vi "Decimate 1D Array.vi"() -> ()   [LabVIEW 2015]
panel:
  out "Acceleration Data - All Channels":dbl[][](graph)
  out "Acceleration Data - Raw Data":dbl[](graph)
  in  "One Channel":dbl[](array[numeric])=[-0.14962495265155748, 0.41037504734844255, 0.7503750473484425, 1.3503750473484426, 0.32358707926196334, 0.8835870792619633, 1.2235870792619634, 1.8235870792619633, 0.5158371040723982, 1.0758371040723982, 1.4158371040723983, 2.015837104072398, 1.0013622642375388, 1.5613622642375389, 1.9013622642375387, 2.501362264237539, 1.2315810460794596, 1.7915810460794597, 2.1315810460794595, 2.7315810460794596, 1.4926225836648097, 2.0526225836648098, 2.3926225836648096, 2.9926225836648097, 1.7403663242081597, 2.30036632420816, 2.6403663242081596, 3.2403663242081597, 2.1837724556787284, 2.7437724556787284, 3.0837724556787283, 3.6837724556787284, 2.4331809540498823, 2.9931809540498824, 3.3331809540498822, 3.9331809540498823, 2.6727105780071363, 3.2327105780071363, 3.572710578007136, 4.172710578007136, 2.7527846546640786, 3.3127846546640787, 3.6527846546640785, 4.252784654664079, 3.199063134137579, 3.759063134137579, 4.099063134137579, 4.699063134137579, 3.383002482831626, 3.943002482831626, 4.283002482831626, 4.8830024828316265, 3.5393424951638277, 4.099342495163828, 4.439342495163828, 5.039342495163828, 3.678036551358494, 4.238036551358494, 4.578036551358494, 5.178036551358494, 3.77794347870013, 4.337943478700129, 4.67794347870013, 5.27794347870013, 3.972363708756191, 4.532363708756192, 4.8723637087561915, 5.472363708756191, 4.209103239125207, 4.769103239125206, 5.109103239125207, 5.709103239125207, 4.28250695958775, 4.84250695958775, 5.182506959587751, 5.78250695958775, 4.408872390322232, 4.9688723903222325, 5.308872390322232, 5.908872390322232, 4.758958504137904, 5.318958504137903, 5.658958504137904, 6.258958504137904, 4.681077878539436, 5.241077878539436, 5.581077878539436, 6.181077878539436, 4.649505296320039, 5.209505296320039, 5.5495052963200395, 6.149505296320039, 4.663003364980422, 5.223003364980421, 5.563003364980422, 6.163003364980422, 4.692743104263729, 5.252743104263729, 5.59274310426373, 6.192743104263729, 4.813363242945864, 5.373363242945864, 5.7133632429458645, 6.313363242945864, 4.8495688944798045, 5.409568894479804, 5.749568894479805, 6.3495688944798045, 4.832958271083728, 5.392958271083728, 5.732958271083729, 6.332958271083728, 4.794309425014819, 5.354309425014819, 5.694309425014819, 6.294309425014819, 4.729519768328653, 5.289519768328653, 5.629519768328653, 6.229519768328653, 4.512270957962928, 5.072270957962928, 5.412270957962928, 6.012270957962928, 4.558016333461781, 5.118016333461782, 5.4580163334617815, 6.058016333461781, 4.373550079676513, 4.933550079676513, 5.273550079676514, 5.873550079676513, 4.205404174649964, 4.765404174649964, 5.105404174649965, 5.705404174649964, 3.9620544887813622, 4.522054488781363, 4.862054488781363, 5.462054488781362, 3.9557536814065983, 4.515753681406599, 4.855753681406599, 5.455753681406598, 3.821833957543013, 4.381833957543013, 4.721833957543013, 5.321833957543014, 3.6260642782488035, 4.186064278248804, 4.526064278248803, 5.126064278248803, 3.3258171871791595, 3.8858171871791596, 4.225817187179159, 4.82581718717916, 3.0319650788286374, 3.5919650788286375, 3.9319650788286373, 4.531965078828637, 2.963344631394424, 3.523344631394424, 3.863344631394424, 4.463344631394424, 2.6667322317798274, 3.2267322317798275, 3.5667322317798273, 4.166732231779827, 2.473099379128181, 3.033099379128181, 3.3730993791281807, 3.973099379128181, 2.192699443858829, 2.752699443858829, 3.092699443858829, 3.692699443858829, 1.7970855115107007, 2.357085511510701, 2.697085511510701, 3.2970855115107005, 1.391362630806126, 1.951362630806126, 2.291362630806126, 2.891362630806126, 1.1947024580658947, 1.7547024580658948, 2.094702458065895, 2.694702458065895, 0.8293390768372463, 1.3893390768372464, 1.7293390768372463, 2.3293390768372464, 0.7165176103423602, 1.2765176103423603, 1.6165176103423602, 2.2165176103423603, 0.21739186152171264, 0.7773918615217127, 1.1173918615217127, 1.7173918615217127, 0.08389711880070679, 0.6438971188007069, 0.9838971188007068, 1.5838971188007067, -0.2014154315838475, 0.35858456841615255, 0.6985845684161525, 1.2985845684161526, -0.45880737655206777, 0.10119262344793228, 0.44119262344793225, 1.0411926234479323, -0.7588321422834481, -0.19883214228344803, 0.14116785771655194, 0.7411678577165519, -1.1726284726040646, -0.6126284726040645, -0.27262847260406453, 0.32737152739593545, -1.530929895098799, -0.970929895098799, -0.630929895098799, -0.030929895098799065, -1.855415216411067, -1.295415216411067, -0.9554152164110671, -0.3554152164110671, -2.1257997826218475, -1.5657997826218475, -1.2257997826218476, -0.6257997826218475, -2.2342862030438306, -1.6742862030438306, -1.3342862030438307, -0.7342862030438306, -2.741606398916626, -2.181606398916626, -1.841606398916626, -1.241606398916626, -2.887792759406135, -2.327792759406135, -1.987792759406135, -1.387792759406135, -3.213592959260521, -2.653592959260521, -2.313592959260521, -1.713592959260521, -3.266690568130646, -2.706690568130646, -2.3666905681306463, -1.7666905681306462, -3.6684175532113046, -3.1084175532113045, -2.7684175532113047, -2.1684175532113046, -3.8842018773676084, -3.3242018773676083, -2.9842018773676084, -2.3842018773676084, -3.7978109000808535, -3.2378109000808535, -2.8978109000808536, -2.2978109000808535, -4.162177095542973, -3.6021770955429733, -3.2621770955429734, -2.6621770955429733, -4.317899007672012, -3.757899007672012, -3.417899007672012, -2.817899007672012, -4.361940882321648, -3.8019408823216483, -3.4619408823216484, -2.8619408823216483, -4.4517483980505705, -3.8917483980505705, -3.5517483980505706, -2.9517483980505705, -4.511118204064262, -3.951118204064262, -3.611118204064262, -3.011118204064262, -4.629422702158851, -4.069422702158851, -3.729422702158851, -3.129422702158851, -4.768299148577401, -4.208299148577401, -3.868299148577401, -3.268299148577401, -4.899995619058348, -4.339995619058348, -3.9999956190583483, -3.3999956190583482, -4.766949699339253, -4.206949699339253, -3.8669496993392527, -3.2669496993392526, -4.859462074009303, -4.299462074009304, -3.9594620740093034, -3.3594620740093033, -4.852682045261981, -4.292682045261982, -3.9526820452619815, -3.3526820452619814, -4.67685667734484, -4.11685667734484, -3.7768566773448398, -3.1768566773448397, -4.690449517396064, -4.130449517396064, -3.790449517396064, -3.190449517396064, -4.8148867377571305, -4.254886737757131, -3.9148867377571306, -3.3148867377571305, -4.582687293451267, -4.022687293451266, -3.682687293451267, -3.082687293451267, -4.543532999964535, -3.983532999964535, -3.643532999964535, -3.043532999964535, -4.31781138883897, -3.7578113888389697, -3.41781138883897, -2.8178113888389698, -4.217078341071507, -3.657078341071507, -3.317078341071507, -2.717078341071507, -4.073221926285143, -3.513221926285143, -3.173221926285143, -2.573221926285143, -3.9650472381739164, -3.4050472381739163, -3.0650472381739164, -2.4650472381739164, -3.8413723612649657, -3.2813723612649657, -2.941372361264966, -2.3413723612649657, -3.617751813992966, -3.057751813992966, -2.717751813992966, -2.117751813992966, -3.342307409185613, -2.782307409185613, -2.442307409185613, -1.8423074091856129, -3.000516474277763, -2.440516474277763, -2.100516474277763, -1.500516474277763, -2.8454216030491355, -2.2854216030491354, -1.9454216030491356, -1.3454216030491355, -2.4517334968884885, -1.8917334968884885, -1.5517334968884886, -0.9517334968884885, -2.260865703872782, -1.7008657038727821, -1.3608657038727823, -0.7608657038727822, -2.1113170451710848, -1.5513170451710847, -1.2113170451710848, -0.6113170451710848, -1.8845857313028413, -1.3245857313028413, -0.9845857313028413, -0.38458573130284135, -1.4514697463196364, -0.8914697463196364, -0.5514697463196364, 0.048530253680363566, -1.2085104708975833, -0.6485104708975833, -0.3085104708975833, 0.29148952910241666, -1.0396797084617442, -0.4796797084617441, -0.13967970846174416, 0.4603202915382558, -0.5479193060350005, 0.012080693964999556, 0.3520806939649995, 0.9520806939649995, -0.30307056326094645, 0.2569294367390536, 0.5969294367390536, 1.1969294367390535]
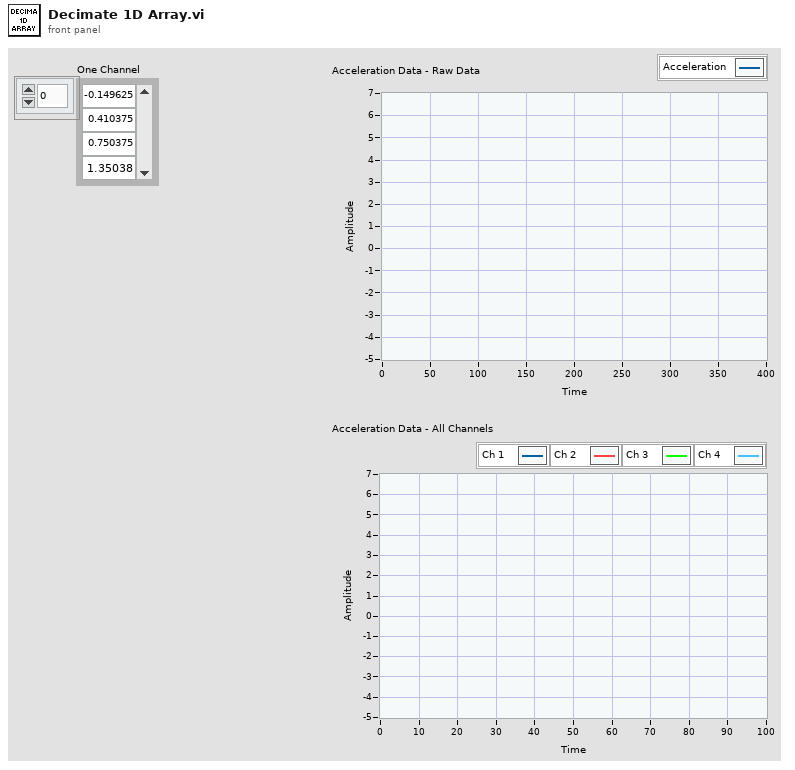
[diagram p1: front panel]
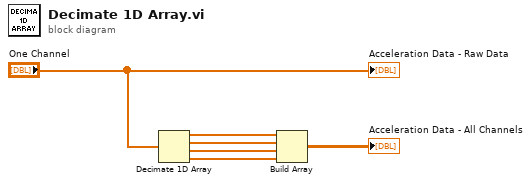
[diagram p0: block diagram]
diagram:
  n1 = Decimate 1D Array "Decimate 1D Array"("One Channel") -> (w3:dbl[], w4:dbl[], w5:dbl[], w2:dbl[])
  n2 = Build Array "Build Array"(w3, w4, w5, w2) -> (→"Acceleration Data - All Channels":dbl[][])
  "Acceleration Data - Raw Data" <- "One Channel"
